vi "Read X-offsets.vi"(8 "error in (no error)":errorcluster, 11 "Configuration in":refnum<class "CV-Configuration.lvclass">) -> (0 "error out":errorcluster, 2 "X-offsets":i32[](array[numeric]), 3 "Configuration out":refnum<class "CV-Configuration.lvclass">)   [LabVIEW 2013, in "CameraVision.lvlib" / "CV-Configuration.lvclass"]
uses:
  CV-Configuration.lvclass
  CV-Configuration.lvclass/CV-Configuration.ctl
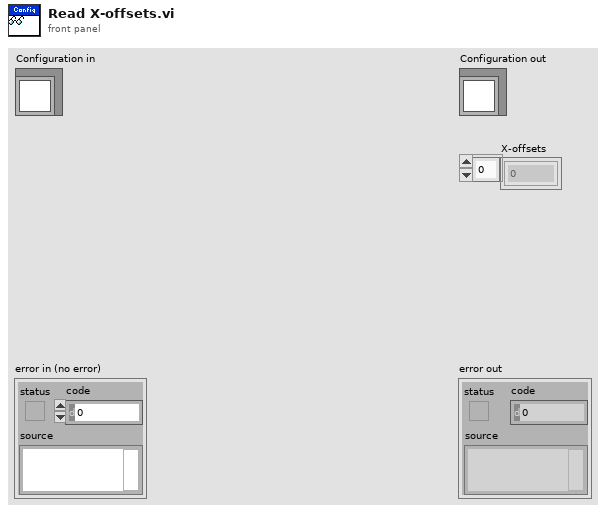
[diagram p1: front panel]
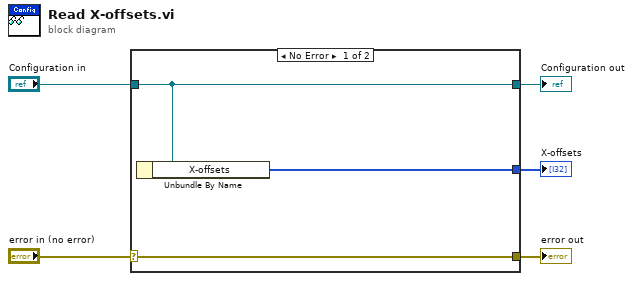
[diagram p0: block diagram]
diagram:
  n1 = case shown="No Error" "error in (no error)" {
    selector: "error in (no error)" -> [w8 w9]
    tunnel: [w8 w9] -> w4
    tunnel: [w7 w10] -> w2
    tunnel: "Configuration in" -> [w7 w10]
    tunnel: [w6 _] -> w1
    frame No Error {
      n2 = Unbundle By Name(w7) -> ("X-offsets"=w6:i32[])
    }
    frame Error {
    }
  }
  "error out" <- w4
  "Configuration out" <- w2
  "X-offsets" <- w1
